vi "Initialize Multi Listbox Column Width.vi"(6 "Popup Listbox":refnum<vi>, 7 "error in (no error)":errorcluster, 10 "Multicolumn Listbox Out":refnum<vi>) -> (0 "error out":errorcluster)   [LabVIEW 2012]
uses:
  <vilib>/Utility/miscctls.llb/LVRowAndColumnTypeDef.ctl
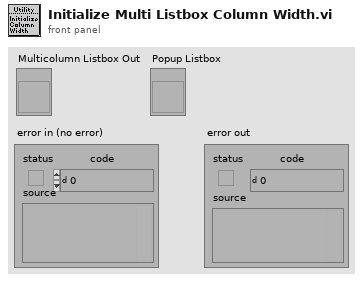
[diagram p1: front panel]
types:
  T1 = typedef "LVRowAndColumnTypeDef.ctl" = cluster{"Row":i32, "Column":i32}
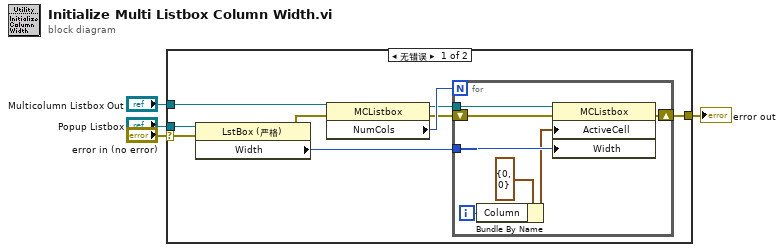
[diagram p0: block diagram]
diagram:
  n1 = case shown="无错误" "error in (no error)" {
    selector: "error in (no error)" -> [w8 w21]
    tunnel: [w7 w21] -> w3
    tunnel: "Popup Listbox" -> [w6 _]
    tunnel: "Multicolumn Listbox Out" -> [w5 _]
    frame No Error {
      n2 = property class="LstBox (严格)"(reference=w6, error in=w8) -> (error out=w10:errorcluster, "Width"=w13:u32)  [unwired: 1 out]
      n3 = property class="MCListbox"(reference=w5, error in=w10) -> (reference out=w11:refnum<vi>, error out=w9:errorcluster, "NumCols"=w12:u32)
      n4 = for {
        N: w12 -> [_]
        tunnel: w13 -> [w20]
        tunnel: w11 -> [w14]
        shift-right: [w15] -> w7
        shift-left: w9 -> [w16]
        i -> [w18]
        n5 = Bundle By Name(cluster=T1 {"Row"=0, "Column"=0} ("Active Cell:Active Cell"), "Column"=w18) -> (w17:T1)
        n6 = property class="MCListbox"(reference=w14, error in=w16, "ActiveCell"=w17, "Width"=w20) -> (error out=w15:errorcluster)  [unwired: 1 out]
      }
    }
    frame Error {
    }
  }
  "error out" <- w3
